vi "enc to inch.vi"(11 "Sensor position":dbl) -> (3 "Inches":dbl)   [LabVIEW 2015]
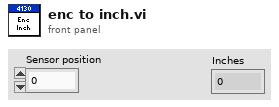
[diagram p1: front panel]
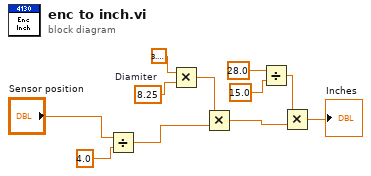
[diagram p0: block diagram]
diagram:
  w11 = 8.25  # Diamiter
  n1 = Divide(x="Sensor position", y=4.0 ("x")) -> (x/y=w2:dbl)
  n2 = Multiply(x=3.141592653589793, y=w11) -> (x*y=w10:dbl)
  n3 = Multiply(x=w10, y=w2) -> (x*y=w5:dbl)
  n4 = Divide(x=28.0, y=15.0) -> (x/y=w6:dbl)
  n5 = Multiply(x=w6, y=w5) -> (x*y=→"Inches":dbl)
